vi "publishWavelength.vi"(8 "error in (no error)":errorcluster, 10 "wavelength":T1, 11 "Monochromator in":refnum<class "Monochromator.lvclass">) -> (0 "error out":errorcluster, 3 "Monochromator out":refnum<class "Monochromator.lvclass">)   [LabVIEW 2016, in "Monochromator.lvclass"]
uses:
  Monochromator.lvclass
  Typedefs/wavelength.ctl
  Monochromator.lvclass/Monochromator.ctl
  MonoPubSubData/MonoPubSubData.lvclass/MonoPubSubData.ctl
  MonoPubSubData/MonoPubSubData.lvclass
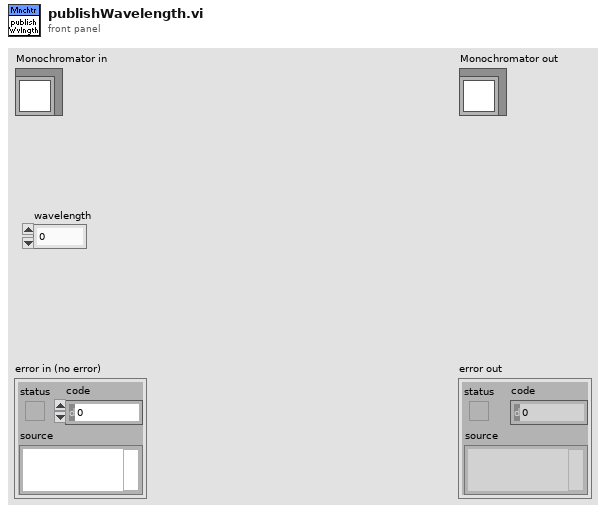
[diagram p1: front panel]
types:
  T1 = typedef "wavelength.ctl" = dbl
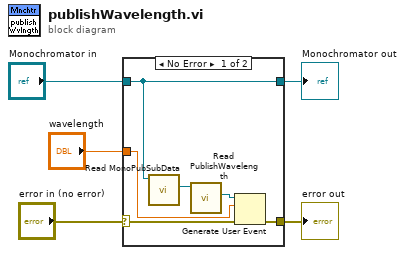
[diagram p0: block diagram]
diagram:
  n1 = case shown="No Error" "error in (no error)" {
    selector: "error in (no error)" -> [w10 w13]
    tunnel: [w9 w13] -> w4
    tunnel: [w8 w12] -> w2
    tunnel: "Monochromator in" -> [w8 w12]
    tunnel: "wavelength" -> [w11 _]
    frame No Error {
      n2 = call "Read MonoPubSubData.vi"("Monochromator in"=w8) -> ("MonoPubSubData.lvclass"=w7:refnum<class "MonoPubSubData.lvclass">)  [unwired: 8 in, 2 out]
      n3 = call "Read PublishWavelength.vi"("MonoPubSubData in"=w7) -> ("PublishWavelength"=w6:refnum<user-event>)  [unwired: 8 in, 2 out]
      n4 = Generate User Event(user event=w6, event data cluster=w11, error in=w10) -> (error out=w9:errorcluster)  [unwired: 1 in, 1 out]
    }
    frame Error {
    }
  }
  "error out" <- w4
  "Monochromator out" <- w2
